vi "advanced_settings.vi"() -> (14 "Radius":dbl, 15 "Amplitude threshold (V)":dbl, 16 "Display resolution":string, 17 "Return":bool, 19 "Firefly mode":bool, 20 "Auto lifetime":bool, 21 "Lower lifetime":dbl, 23 "Stereomode":bool, 24 "Upper lifetime":dbl, 25 "ANSI limit":dbl, 26 "Pentero mode":bool, 27 "Channel":dbl)   [LabVIEW 2020]
panel:
  in  "Quit":bool
  in  "Save":bool
  in  "Display settings":T1={"Lower lifetime"=3.0, "Upper lifetime"=6.0, "Channel"=2.0, "ANSI limit"=20.0, "Auto lifetime"=FALSE, "Threshold (V)"=0.05, "Stereomode"=FALSE, "Firefly camera"=TRUE, "Radius"=1.0, "Pentero mode"=FALSE} {"Radius" min=0.0 max=1.0 step=0.1; "ANSI limit" min=1.0 max=100.0 step=1.0; "Channel" min=1.0 max=4.0 step=1.0; "Upper lifetime" min=2.0 max=10.0 step=1.0; "Lower lifetime" min=1.0 max=6.0 step=1.0}
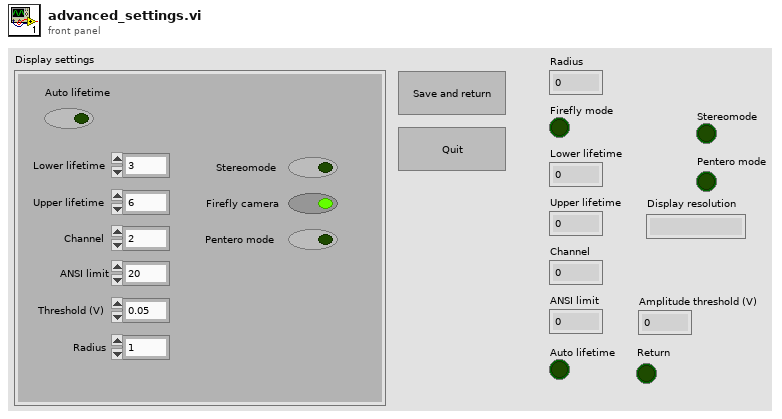
[diagram p1: front panel]
types:
  T1 = cluster{"Lower lifetime":dbl, "Upper lifetime":dbl, "Channel":dbl, "ANSI limit":dbl, "Auto lifetime":bool, "Threshold (V)":dbl, "Stereomode":bool, "Firefly camera":bool, "Radius":dbl, "Pentero mode":bool}
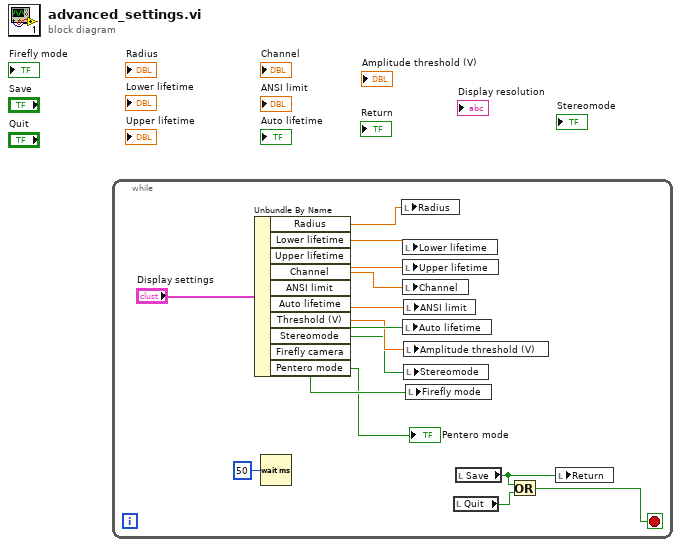
[diagram p0: block diagram]
diagram:
  n1 = while {
    stop <- w13 stop-if-true
    n2 = Unbundle By Name("Display settings") -> ("Radius"=w5:dbl, "Lower lifetime"=w12:dbl, "Upper lifetime"=w11:dbl, "Channel"=w10:dbl, "ANSI limit"=w9:dbl, "Auto lifetime"=w8:bool, "Threshold (V)"=w6:dbl, "Stereomode"=w4:bool, "Firefly camera"=w3:bool, "Pentero mode"=→"Pentero mode":bool)
    n3 = Wait (ms)(milliseconds to wait=u32 50) -> ()  [unwired: 1 out]
    n4 = local write "Radius"(w5) -> ()
    n5 = local write "Lower lifetime"(w12) -> ()
    n6 = local write "Upper lifetime"(w11) -> ()
    n7 = local write "Channel"(w10) -> ()
    n8 = local write "Auto lifetime"(w8) -> ()
    n9 = local write "ANSI limit"(w9) -> ()
    n10 = local write "Amplitude threshold (V)"(w6) -> ()
    n11 = local write "Stereomode"(w4) -> ()
    n12 = local write "Firefly mode"(w3) -> ()
    n13 = local read "Quit"() -> (w14:bool)
    n14 = local read "Save"() -> (w7:bool)
    n15 = Or(x=w7, y=w14) -> (x .or. y?=w13:bool)
    n16 = local write "Return"(w7) -> ()
  }
